vi "Home Screen.vi"() -> ()   [LabVIEW 2025]
doc: "Login"
uses:
  Host Globals/Global 1.vi
panel:
  out "Time":string
  out "User":string
  in  "Administration":bool
  in  "Audit Trail":bool
  in  "Exit":bool
  in  "HistoricalData":bool
  in  "ConfigurationMain":bool
  in  "Maintenance":bool
  in  "Test":bool
  # "Automated Testing of NVH Powertrain Lab"
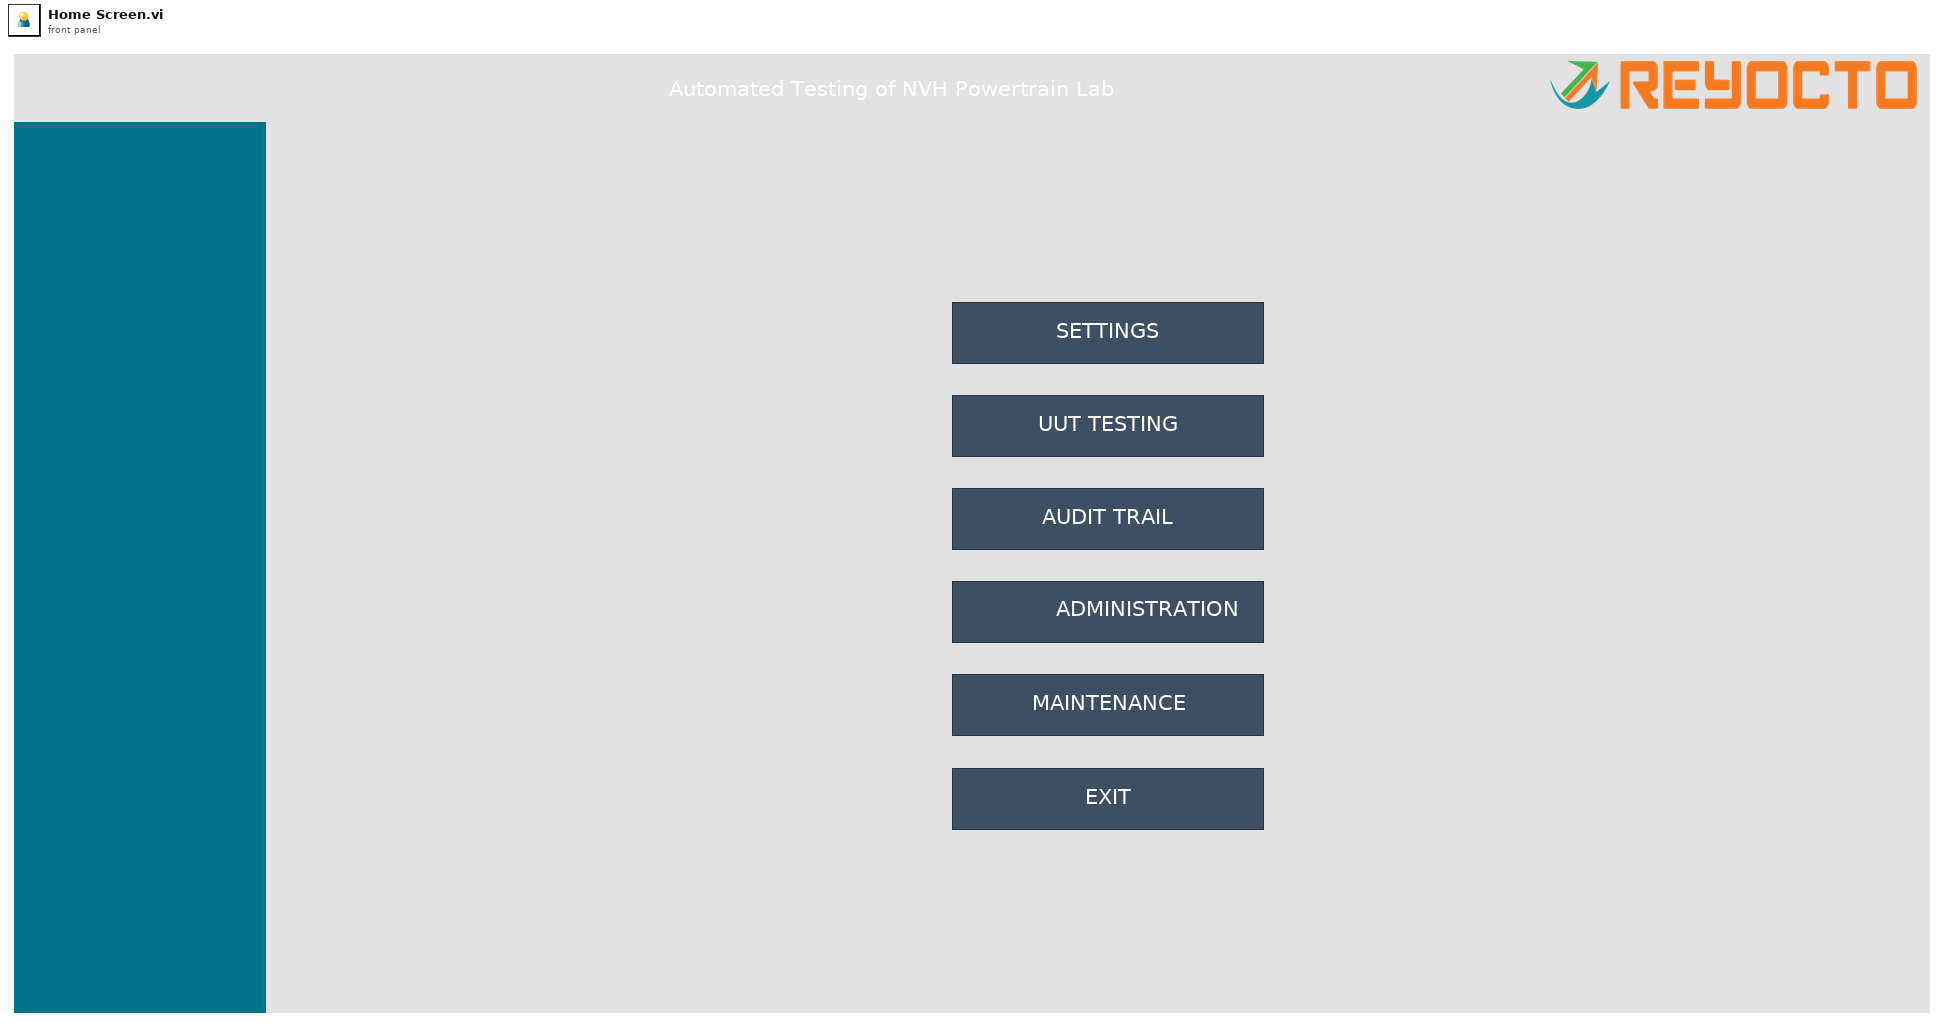
[diagram p1: front panel]
types:
  T1 = enum32{"Invalid", "Standard", "Closed", "Hidden", "Minimized", "Maximized"}
  T2 = enum32{"invalid app kind", "Development System", "Run Time System", "Student Edition", "Embedded LabVIEW", "Evaluation", "Custom"}
  T3 = cluster{"Core":cluster{"Current VI Reference":refnum<vi>, "Close Panel on Exit?":bool}, "VI Path":path, "Your string data":string}
  T4 = cluster{"Current VI Reference":refnum<vi>, "Close Panel on Exit?":bool}
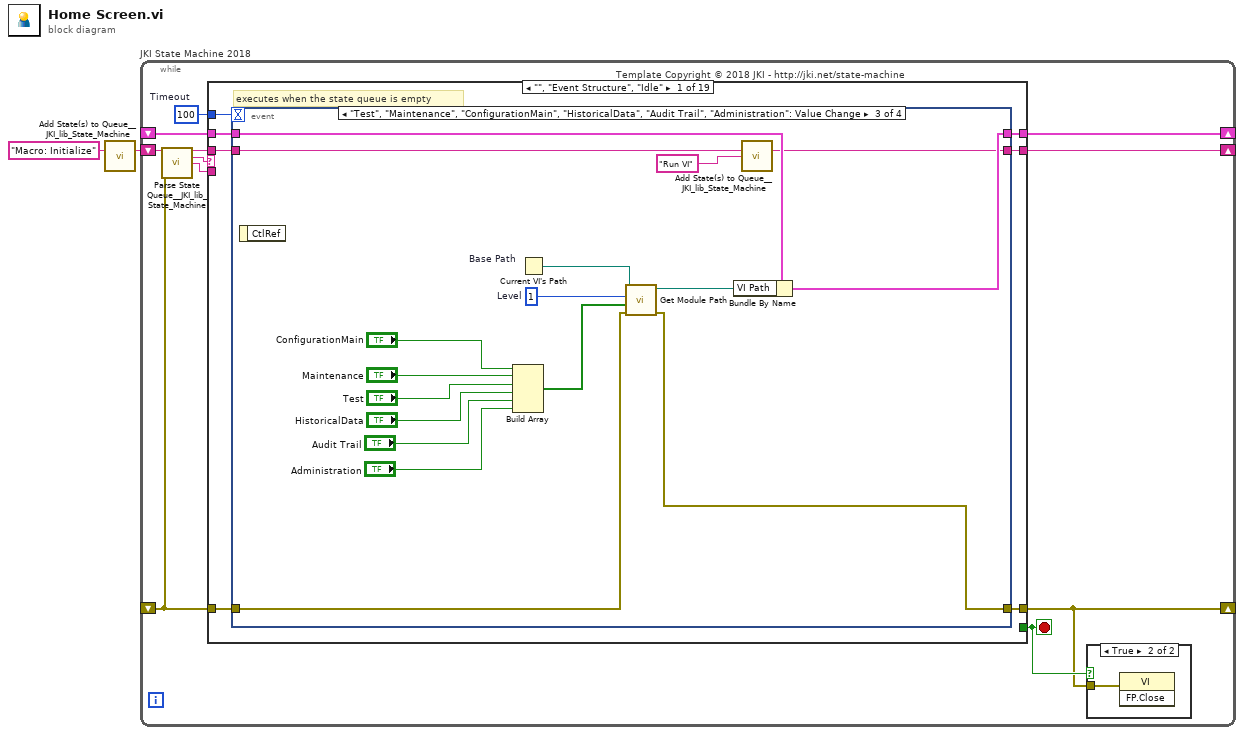
[diagram p0: block diagram]
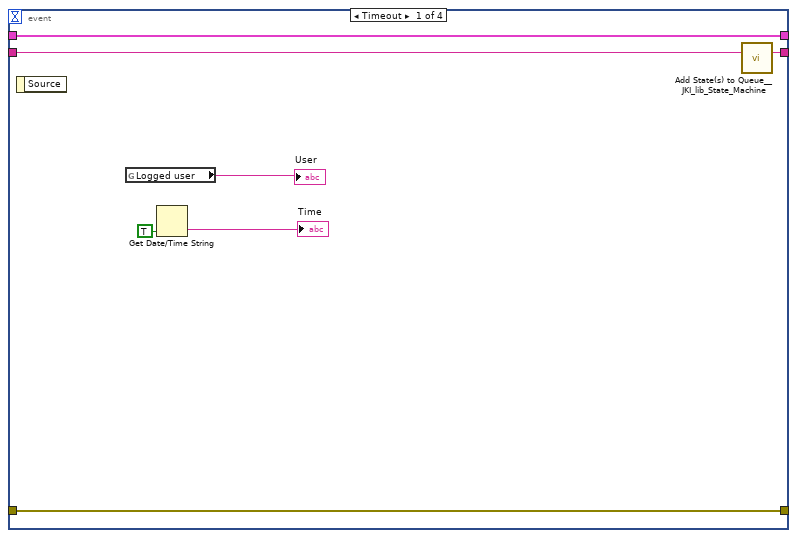
[diagram p3: hidden frame]
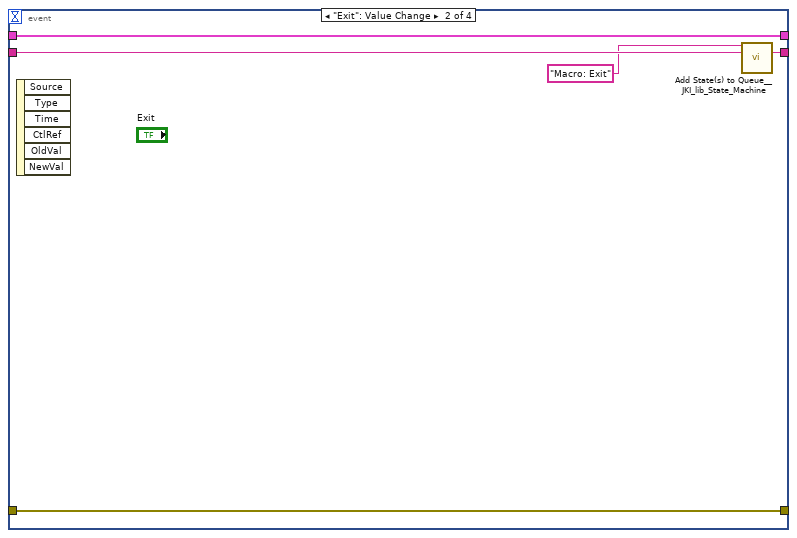
[diagram p4: hidden frame]
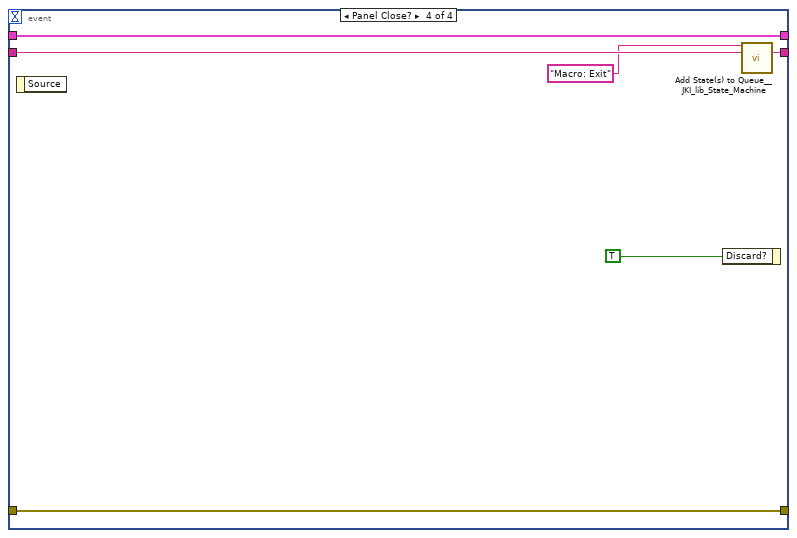
[diagram p5: hidden frame]
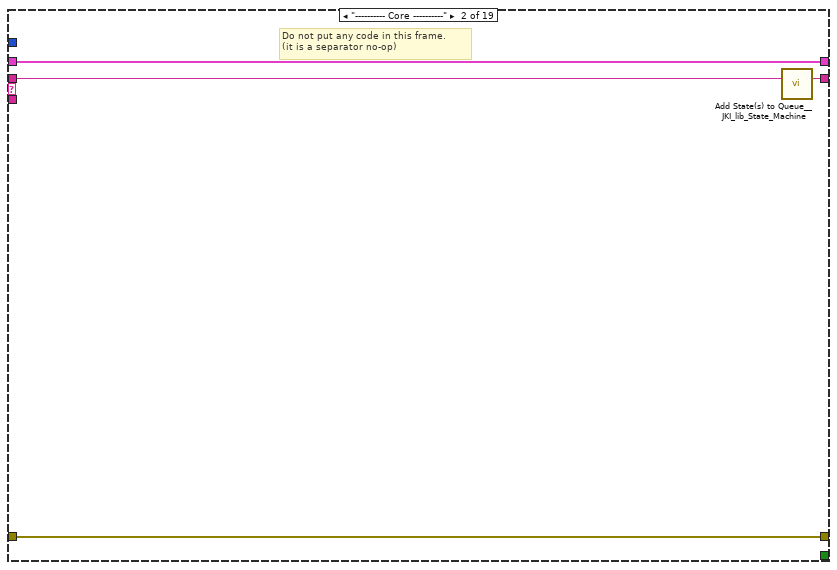
[diagram p6: hidden frame]
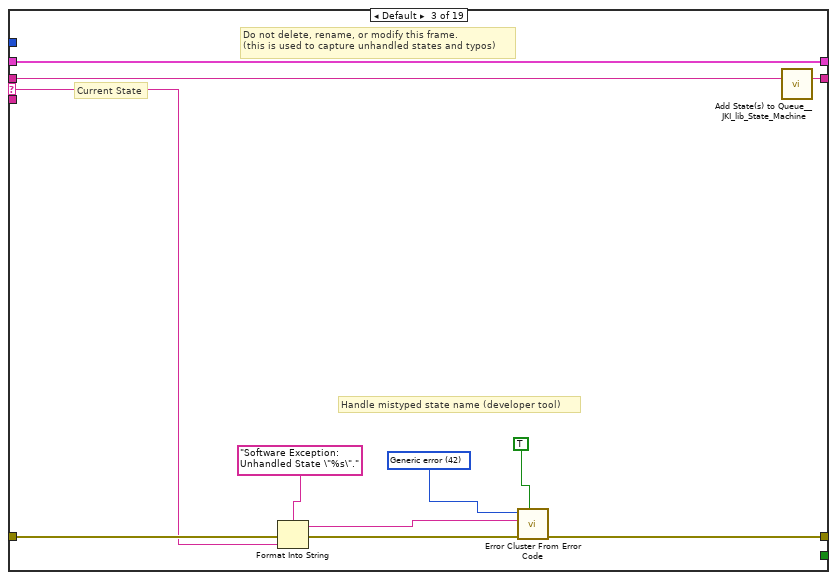
[diagram p7: hidden frame]
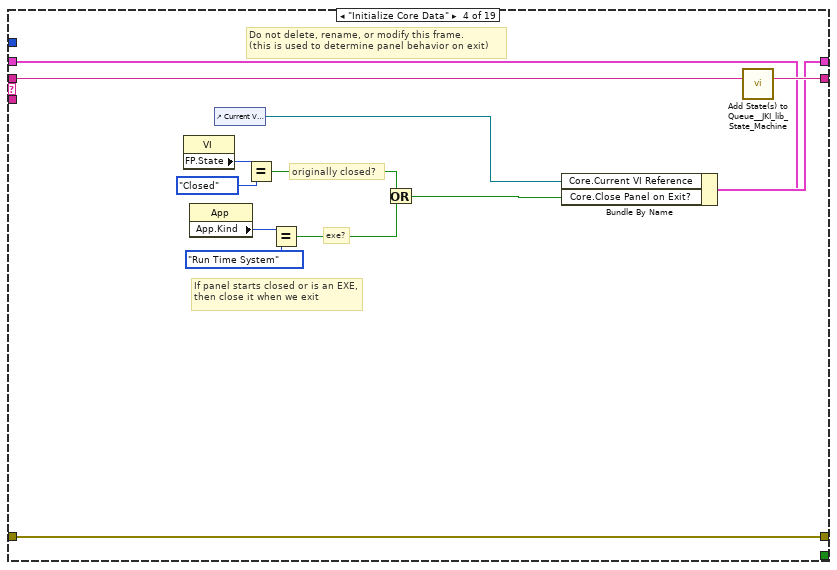
[diagram p8: hidden frame]
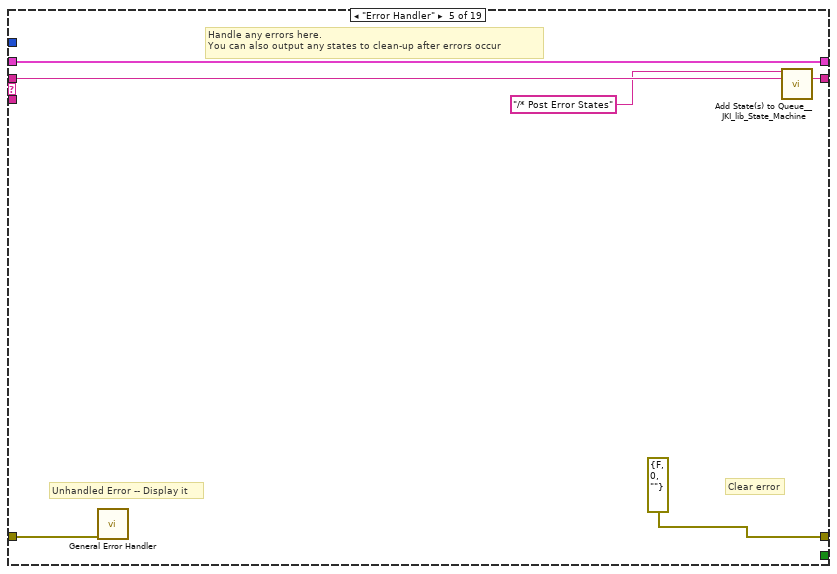
[diagram p9: hidden frame]
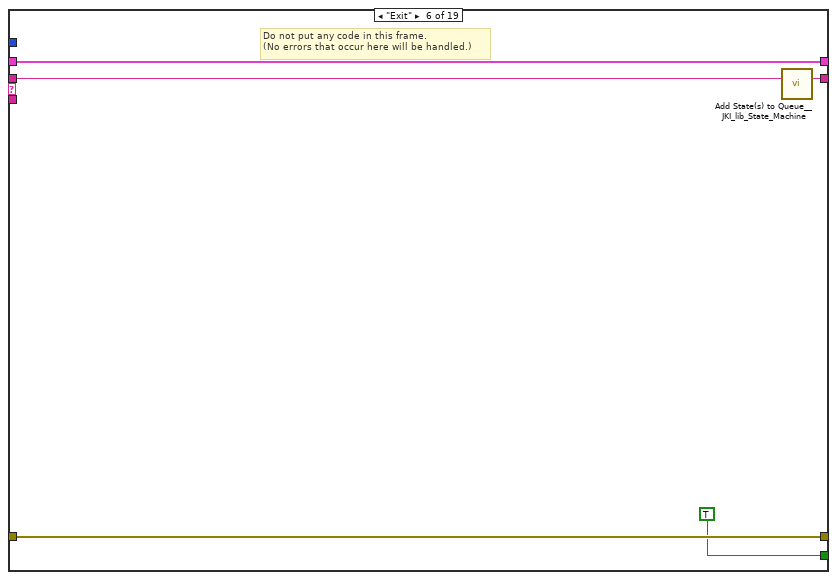
[diagram p10: hidden frame]
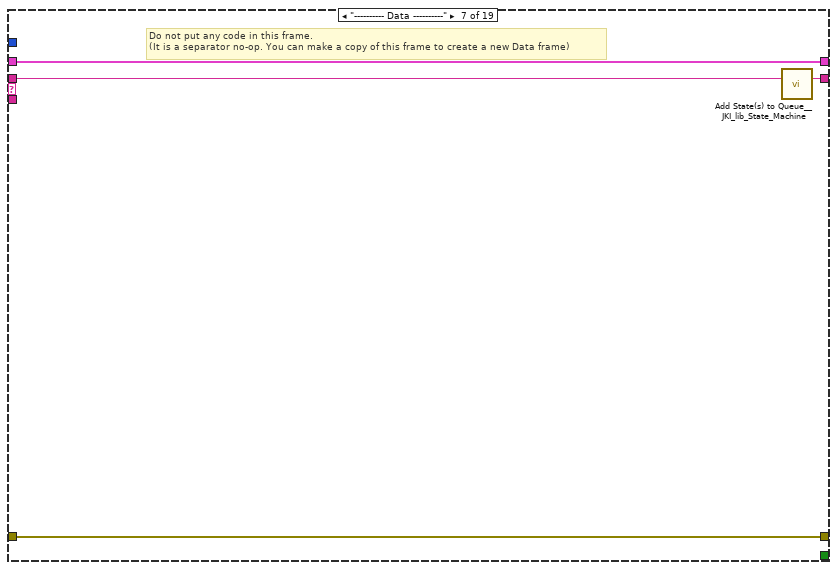
[diagram p11: hidden frame]
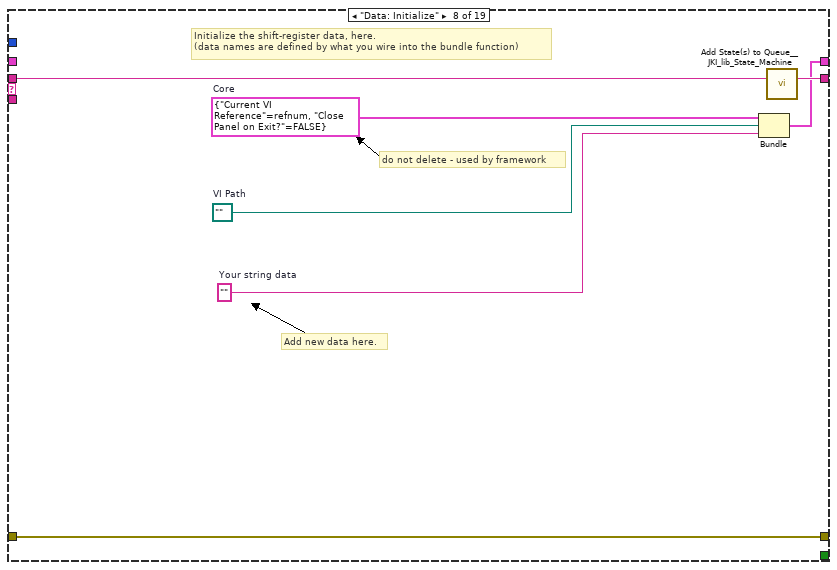
[diagram p12: hidden frame]
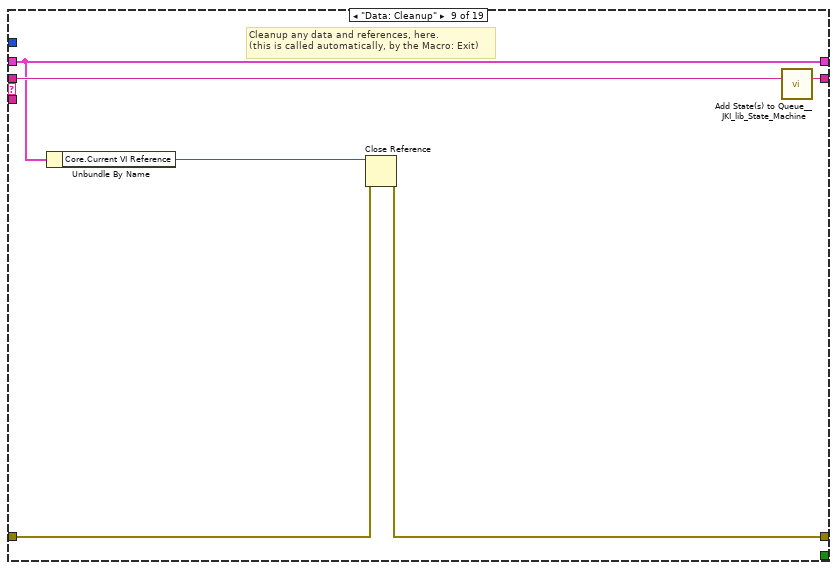
[diagram p13: hidden frame]
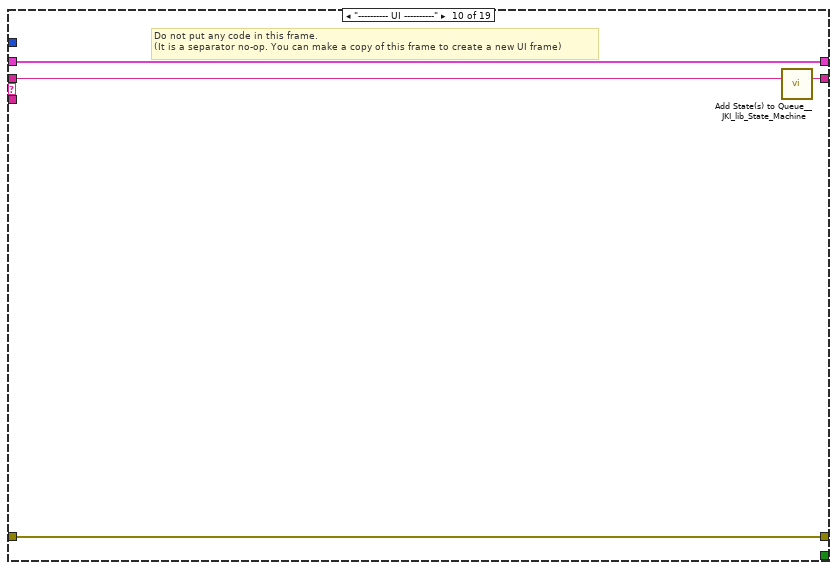
[diagram p14: hidden frame]
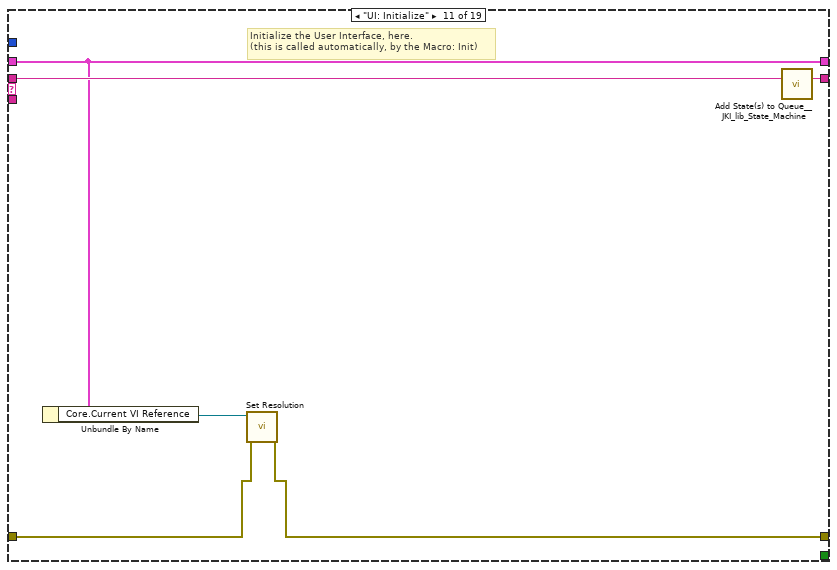
[diagram p15: hidden frame]
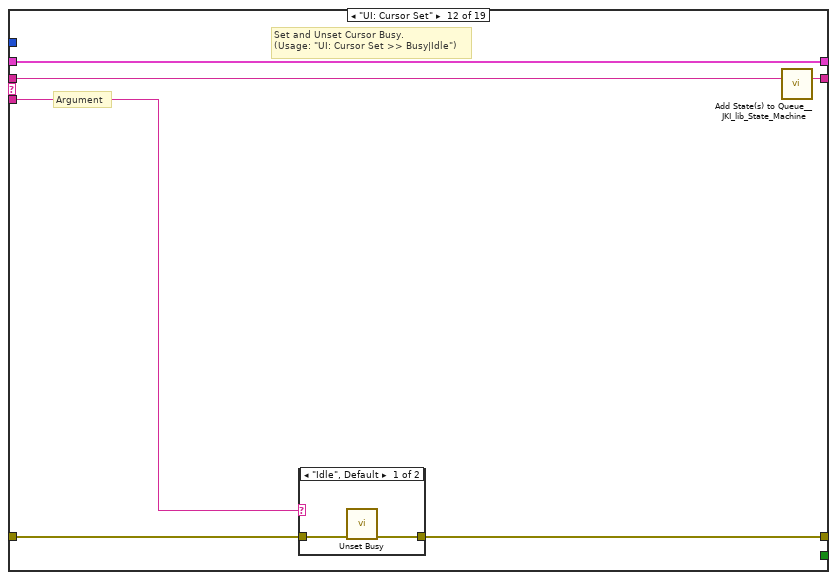
[diagram p16: hidden frame]
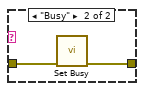
[diagram p17: hidden frame]
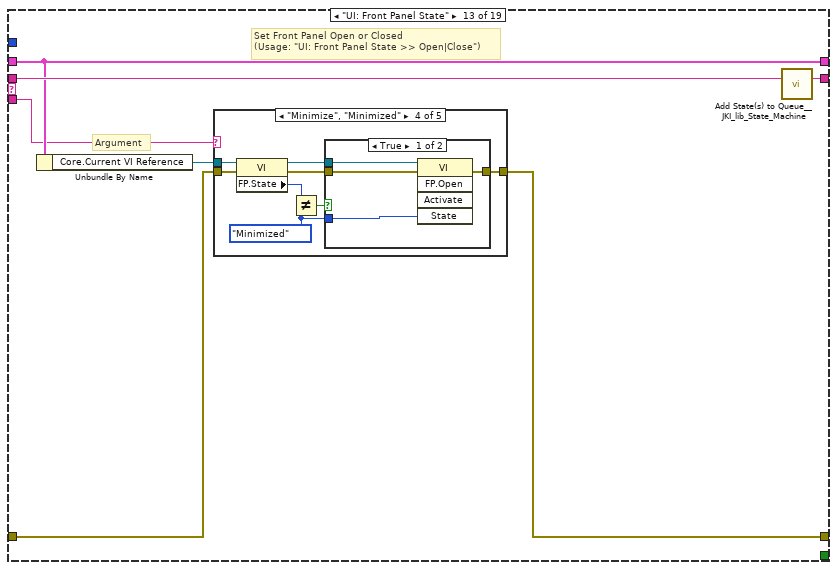
[diagram p18: hidden frame]
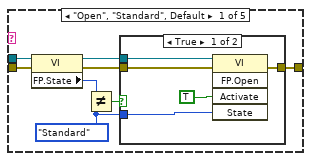
[diagram p19: hidden frame]
diagram:
  n1 = call <vilib>:"Add State(s) to Queue__JKI_lib_State_Machine.vi"("State(s) in (\"\")"="Macro: Initialize") -> ("States Out"=w2:string)  [unwired: 14 in]
  n2 = while "JKI State Machine 2018" {
    shift-right: [w8] -> _
    shift-left: _ -> [w7]
    shift-right: [w3] -> _
    shift-left: _ -> [w5]
    shift-right: [w9] -> _
    shift-left: w2 -> [w10]
    stop <- w4 stop-if-true
    w6 = 100  # Timeout
    # "Template Copyright © 2018 JKI - http://jki.net/state-machine"
    n3 = call <vilib>:"Parse State Queue__JKI_lib_State_Machine.vi"("State Queue"=w10, "Error In (no error)"=w5) -> ("Remaining States"=w12:string, "Current State"=w13:string, "Arguments"=w11:string)  [unwired: 11 in]
    n4 = case shown="\"\", \"Event Structure\", \"Idle\"" w13 {
      selector: w13 -> [_ _ w61 _ _ _ _ _ _ _ _ _ _ _ _ _ _ _ _]
      tunnel: w12 -> [w21 w60 w65 w84 w90 w95 w99 w106 w112 w116 w122 w128 w139 w208 w213 w223 w227 w240 w253]
      tunnel: w11 -> [_ _ _ _ _ _ _ _ _ _ _ w123 w133 _ _ _ _ _ _]
      tunnel: w7 -> [w19 w57 w63 w77 w87 w93 w96 _ w107 w113 w118 w126 w135 w205 w210 w220 w224 w237 w250]
      tunnel: [w18 w58 w67 w81 errorcluster {"status"=FALSE, "code"=0, "source"=""} ("error out") w92 w97 w103 w108 w114 w119 w124 w136 w206 w211 w221 w225 w229 w251] -> w3
      tunnel: w5 -> [w17 w58 w66 w81 w86 w92 w97 w103 w109 w114 w120 w125 w137 w206 w211 w221 w225 w238 w251]
      tunnel: [w20 w59 w64 w83 w89 w94 w98 w105 w111 w115 w121 w127 w138 w207 w212 w222 w226 w239 w252] -> w9
      tunnel: [_ _ _ _ _ TRUE _ _ _ _ _ _ _ _ _ _ _ w228 _] -> w4
      tunnel: [w16 w57 w63 w82 w87 w93 w96 w104 w107 w113 w118 w126 w135 w205 w210 w220 w224 w237 w250] -> w8
      tunnel: w6 -> [w15 _ _ _ _ _ _ _ _ _ _ _ _ _ _ _ _ _ _]
      frame "", "Event Structure", "Idle" {
        # "executes when the state queue is empty"
        n5 = event shown="[2] \"Test\", \"Maintenance\", \"ConfigurationMain\", \"HistoricalData\", \"Audit Trail\", \"Administration\": Value Change" {
          selector: _ -> [_ _ _ _]
          dyn-events: _ -> [_ _ _ _]
          timeout: w15 -> [_ _ _ _]
          tunnel: w21 -> [w28 w33 w39 w56]
          tunnel: [w27 w32 w40 w55] -> w20
          tunnel: w19 -> [w25 w30 w43 w53]
          tunnel: [w26 w31 w34 w54] -> w18
          tunnel: w17 -> [w26 w31 w45 w54]
          tunnel: [w25 w30 w42 w53] -> w16
          event Timeout {
            n6 = event-data() -> ()  [unwired: 1 in, 1 out]
            n7 = global read "Global 1.vi" "Logged user"() -> (→"User":string)
            n8 = Get Date/Time String(want seconds? (F)=TRUE) -> (time string=→"Time":string)  [unwired: 2 in, 1 out]
            n9 = call <vilib>:"Add State(s) to Queue__JKI_lib_State_Machine.vi"("State(s) in (\"\")"=w28) -> ("States Out"=w27:string)  [unwired: 14 in]
          }
          event "Exit": Value Change {
            n10 = event-data() -> ()  [unwired: 1 in, 6 out]
            n11 = call <vilib>:"Add State(s) to Queue__JKI_lib_State_Machine.vi"("State(s) in Front (\"\")"="Macro: Exit", "State(s) in (\"\")"=w33) -> ("States Out"=w32:string)  [unwired: 13 in]
          }
          event "Test", "Maintenance", "ConfigurationMain", "HistoricalData", "Audit Trail", "Administration": Value Change {
            w46 = 1  # Level
            n12 = event-data() -> ()  [unwired: 1 in, 1 out]
            n13 = Build Array("ConfigurationMain", "Maintenance", "Test", "HistoricalData", "Audit Trail", "Administration") -> (w44:bool[])
            n14 = Current VI's Path "Base Path"() -> (path=w47:path)
            n15 = call "Get Module Path.vi"("error in (no error)"=w45, "Array 2"=w44, "Level"=w46, "path"=w47) -> ("error out"=w34:errorcluster, "Selected Path"=w41:path)  [unwired: 5 in, 1 out]
            n16 = Bundle By Name(cluster=w43, "VI Path"=w41) -> (w42:T3)
            n17 = call <vilib>:"Add State(s) to Queue__JKI_lib_State_Machine.vi"("State(s) in (\"\")"=w39, "State(s) at Back (\"\")"="Run VI" ("State(s) at Back (\"\")")) -> ("States Out"=w40:string)  [unwired: 13 in]
          }
          event Panel Close? {
            n18 = event-data() -> ()  [unwired: 1 in, 1 out]
            n19 = event-data("Discard?"=TRUE) -> ()  [unwired: 1 in, 1 out]
            n20 = call <vilib>:"Add State(s) to Queue__JKI_lib_State_Machine.vi"("State(s) in Front (\"\")"="Macro: Exit", "State(s) in (\"\")"=w56) -> ("States Out"=w55:string)  [unwired: 13 in]
          }
        }
      }
      frame "---------- Core ----------" {
        # "Do not put any code in this frame.\n(it is a separator no-op)"
        n21 = call <vilib>:"Add State(s) to Queue__JKI_lib_State_Machine.vi"("State(s) in (\"\")"=w60) -> ("States Out"=w59:string)  [unwired: 14 in]
      }
      frame Default {
        w70 = 42 items=["No error", "Argument error", "Memory is full", "Out of zone", "End of file", "File already open", "Generic file I/O error", "File not found", "File permission error", "Disk is full", "Duplicate path", "Too many files open", "System feature not enabled", "Resource file not found", "Cannot add resource", "Resource not found", "Image not found", "Image memory error", "Pen does not exist", "Config type invalid", "Config token not found", "Config parse error", "Config memory error", "Bad external code format", "Bad external code offset", "External code not present", "Null window", "Destroy window error", "Null menu", "Print aborted", "Bad print record", "Print driver error", "Windows error during printing", "Memory error during printing", "Print dialog error", "Generic print error", "Invalid device refnum", "Device not found", "Device parameter error", "Device unit error", "Cannot open device", "Device call aborted", "Generic error", "Cancelled by user", "Object ID too low", "Object ID too high", "Object not in heap", "Unknown heap", "Unknown object (invalid DefProc)", "Unknown object (DefProc not in table)", "Message out of range", "Invalid (null) method", "Unknown message", "Manager call not supported", "Bad address", "Network operation in progress", "Network operation timed out", "Connection is busy", "Network attribute not supported", "Network error", "Address in use", "System out of memory", "Connection aborted", "Connection refused", "Not connected", "Already connected", "Connection closed", "Initialization error (interapplication manager)", "Bad occurrence", "Wait on unbound occurrence handler", "Occurrence queue overflow", "Datalog type conflict", "Unused", "Unrecognized type (interapplication manager)", "Memory corrupt", "Failed to make temporary DLL", "Old CIN version", "Drag socket not found", "Failed to load drop-object", "Failed to register OLE object", "Failed to release OLE object", "Format specifier type mismatch", "Unknown format specifier", "Too few format specifiers", "Too many format specifiers", "Scan failed", "Newer CIN version", "Error converting to variant", "Runtime menu error", "Password tampered", "Variant attribute not found", "Incompatible variant data type", "Event data is not available", "Event Store is not present", "Occurrence is not found", "Event Queue is not created", "Event info is not available", "Refnum passed is NULL", "Error retrieving Class GUID", "Error retrieving CoClass GUID", "Error retrieving TypeLib GUID.", "Bad built application magic bytes.", "Specific driver is different from the specific driver associated with the Logical Name.", "There is no session opened to the class driver.", "Max Error", "MAX - Error with config objects", "MAX - Error loading configuration", "MAX - Group not supported"]
        # "Current State"
        # "Do not delete, rename, or modify this frame.\n(this is used to capture unhandled states and typos)"
        # "Handle mistyped state name (developer tool)"
        n22 = Format Into String(format string="Software Exception: Unhandled State \"%s\"." ("message"), error in=w66, w61) -> (resulting string=w69:string, error out=w68:errorcluster)  [unwired: 1 in]
        n23 = call <vilib>:"Error Cluster From Error Code.vi"("show call chain? (False)"=TRUE, "error in (no error)"=w68, "error message (\"\")"=w69, "error code (0)"=w70) -> ("error out"=w67:errorcluster)  [unwired: 5 in]
        n24 = call <vilib>:"Add State(s) to Queue__JKI_lib_State_Machine.vi"("State(s) in (\"\")"=w65) -> ("States Out"=w64:string)  [unwired: 14 in]
      }
      frame "Initialize Core Data" {
        # "Do not delete, rename, or modify this frame.\n(this is used to determine panel behavior on exit)"
        # "originally closed?"
        # "exe?"
        # "If panel starts closed or is an EXE, then close it when we exit"
        n25 = property class="VI"() -> ("FP.State"=w74:T1)  [unwired: 2 in, 2 out]
        n26 = property class="App"() -> ("App.Kind"=w80:T2)  [unwired: 2 in, 2 out]
        n27 = control-ref of="Current VI Reference"() -> (w75:refnum<vi>)
        n28 = Equal?(x=w74, y=T1."Closed" ("Front Panel Window:State")) -> (x = y?=w72:bool)
        n29 = Equal?(x=w80, y=T2."Run Time System" ("Application:Kind")) -> (x = y?=w78:bool)
        n30 = Or(x=w72, y=w78) -> (x .or. y?=w76:bool)
        n31 = Bundle By Name(cluster=w77, "Core.Current VI Reference"=w75, "Core.Close Panel on Exit?"=w76) -> (w82:T3)
        n32 = call <vilib>:"Add State(s) to Queue__JKI_lib_State_Machine.vi"("State(s) in (\"\")"=w84) -> ("States Out"=w83:string)  [unwired: 14 in]
      }
      frame "Error Handler" {
        # "Unhandled Error -- Display it"
        # "Handle any errors here.\nYou can also output any states to clean-up after errors occur"
        # "Clear error"
        n33 = call <vilib>:"General Error Handler.vi"("error in (no error)"=w86) -> ()  [unwired: 10 in, 5 out]
        n34 = call <vilib>:"Add State(s) to Queue__JKI_lib_State_Machine.vi"("State(s) in Front (\"\")"="/* Post Error States", "State(s) in (\"\")"=w90) -> ("States Out"=w89:string)  [unwired: 13 in]
      }
      frame "Exit" {
        # "Do not put any code in this frame.\n(No errors that occur here will be handled.)"
        n35 = call <vilib>:"Add State(s) to Queue__JKI_lib_State_Machine.vi"("State(s) in (\"\")"=w95) -> ("States Out"=w94:string)  [unwired: 14 in]
      }
      frame "---------- Data ----------" {
        # "Do not put any code in this frame.\n(It is a separator no-op. You can make a copy of this frame to create a new Data frame)"
        n36 = call <vilib>:"Add State(s) to Queue__JKI_lib_State_Machine.vi"("State(s) in (\"\")"=w99) -> ("States Out"=w98:string)  [unwired: 14 in]
      }
      frame "Data: Initialize" {
        w100 = path ""  # VI Path
        w101 = T4 {"Current VI Reference"=refnum, "Close Panel on Exit?"=FALSE}  # Core
        w102 = ""  # Your string data
        # "do not delete - used by framework"
        # "Add new data here."
        # "Initialize the shift-register data, here.\n(data names are defined by what you wire into the bundle function)"
        n37 = Bundle("Core"=w101, "VI Path"=w100, "Your string data"=w102) -> (w104:T3)  [unwired: 1 in]
        n38 = call <vilib>:"Add State(s) to Queue__JKI_lib_State_Machine.vi"("State(s) in (\"\")"=w106) -> ("States Out"=w105:string)  [unwired: 14 in]
      }
      frame "Data: Cleanup" {
        # "Cleanup any data and references, here.\n(this is called automatically, by the Macro: Exit)"
        n39 = Unbundle By Name(w107) -> ("Core.Current VI Reference"=w110:refnum<vi>)
        n40 = Close Reference(reference=w110, error in (no error)=w109) -> (error out=w108:errorcluster)
        n41 = call <vilib>:"Add State(s) to Queue__JKI_lib_State_Machine.vi"("State(s) in (\"\")"=w112) -> ("States Out"=w111:string)  [unwired: 14 in]
      }
      frame "---------- UI ----------" {
        # "Do not put any code in this frame.\n(It is a separator no-op. You can make a copy of this frame to create a new UI frame)"
        n42 = call <vilib>:"Add State(s) to Queue__JKI_lib_State_Machine.vi"("State(s) in (\"\")"=w116) -> ("States Out"=w115:string)  [unwired: 14 in]
      }
      frame "UI: Initialize" {
        # "Initialize the User Interface, here.\n(this is called automatically, by the Macro: Init)"
        n43 = Unbundle By Name(w118) -> ("Core.Current VI Reference"=w117:refnum<vi>)
        n44 = call "Set Resolution.vi"("error in (no error)"=w120, "VI in"=w117) -> ("error out"=w119:errorcluster)  [unwired: 8 in, 1 out]
        n45 = call <vilib>:"Add State(s) to Queue__JKI_lib_State_Machine.vi"("State(s) in (\"\")"=w122) -> ("States Out"=w121:string)  [unwired: 14 in]
      }
      frame "UI: Cursor Set" {
        # "Argument"
        # "Set and Unset Cursor Busy.\n(Usage: \"UI: Cursor Set >> Busy|Idle\")"
        n46 = case shown="\"Idle\", Default" w123 {
          tunnel: w125 -> [w130 w132]
          tunnel: [w129 w131] -> w124
          frame "Idle", Default {
            n47 = call <vilib>:"Unset Busy.vi"("error in (no error)"=w130) -> ("error out"=w129:errorcluster)  [unwired: 10 in]
          }
          frame "Busy" {
            n48 = call <vilib>:"Set Busy.vi"("error in (no error)"=w132) -> ("error out"=w131:errorcluster)  [unwired: 9 in, 1 out]
          }
        }
        n49 = call <vilib>:"Add State(s) to Queue__JKI_lib_State_Machine.vi"("State(s) in (\"\")"=w128) -> ("States Out"=w127:string)  [unwired: 14 in]
      }
      frame "UI: Front Panel State" {
        # "Argument"
        # "Set Front Panel Open or Closed\n(Usage: \"UI: Front Panel State >> Open|Close\")"
        n50 = Unbundle By Name(w135) -> ("Core.Current VI Reference"=w134:refnum<vi>)
        n51 = case shown="\"Minimize\", \"Minimized\"" w133 {
          tunnel: w137 -> [w145 w160 w171 w184 w197]
          tunnel: [w147 w161 w173 w186 w199] -> w136
          tunnel: w134 -> [w146 w158 w172 w185 w198]
          frame "Open", "Standard", Default {
            w140 = T1."Standard" ("State")
            n52 = property class="VI"(reference=w146, error in=w145) -> (reference out=w143:refnum<vi>, error out=w144:errorcluster, "FP.State"=w142:T1)
            n53 = Not Equal?(x=w142, y=w140) -> (x != y?=w141:bool)
            n54 = case shown="True" w141 {
              tunnel: [w151 w153] -> w147
              tunnel: w144 -> [w150 w153]
              tunnel: w143 -> [w149 _]
              tunnel: w140 -> [w148 _]
              frame True {
                n55 = invoke class="VI" method="FP.Open"(reference=w149, error in=w150, "Activate"=TRUE, "State"=w148) -> (error out=w151:errorcluster)  [unwired: 1 in, 4 out]
              }
              frame False {
              }
            }
          }
          frame "Close", "Closed" {
            n56 = property class="VI"(reference=w158, error in=w160) -> (reference out=w157:refnum<vi>, error out=w159:errorcluster, "FP.State"=w155:T1)
            n57 = Not Equal?(x=w155, y=T1."Closed" ("Front Panel Window:State")) -> (x != y?=w154:bool)
            n58 = case shown="True" w154 {
              tunnel: [w162 w165] -> w161
              tunnel: w159 -> [w162 w164]
              tunnel: w157 -> [_ w163]
              frame False {
              }
              frame True {
                n59 = invoke class="VI" method="FP.Close"(reference=w163, error in=w164) -> (error out=w165:errorcluster)  [unwired: 1 in, 2 out]
              }
            }
          }
          frame "Hidden", "Hide" {
            w166 = T1."Hidden" ("State")
            n60 = property class="VI"(reference=w172, error in=w171) -> (reference out=w169:refnum<vi>, error out=w170:errorcluster, "FP.State"=w168:T1)
            n61 = Not Equal?(x=w168, y=w166) -> (x != y?=w167:bool)
            n62 = case shown="True" w167 {
              tunnel: [w177 w178] -> w173
              tunnel: w170 -> [w176 w178]
              tunnel: w169 -> [w175 _]
              tunnel: w166 -> [w174 _]
              frame True {
                n63 = invoke class="VI" method="FP.Open"(reference=w175, error in=w176, "State"=w174) -> (error out=w177:errorcluster)  [unwired: 2 in, 4 out]
              }
              frame False {
              }
            }
          }
          frame "Minimize", "Minimized" {
            w179 = T1."Minimized" ("State")
            n64 = property class="VI"(reference=w185, error in=w184) -> (reference out=w182:refnum<vi>, error out=w183:errorcluster, "FP.State"=w181:T1)
            n65 = Not Equal?(x=w181, y=w179) -> (x != y?=w180:bool)
            n66 = case shown="True" w180 {
              tunnel: [w190 w191] -> w186
              tunnel: w183 -> [w189 w191]
              tunnel: w182 -> [w188 _]
              tunnel: w179 -> [w187 _]
              frame True {
                n67 = invoke class="VI" method="FP.Open"(reference=w188, error in=w189, "State"=w187) -> (error out=w190:errorcluster)  [unwired: 2 in, 4 out]
              }
              frame False {
              }
            }
          }
          frame "Maximize", "Maximized" {
            w192 = T1."Maximized" ("State")
            n68 = property class="VI"(reference=w198, error in=w197) -> (reference out=w195:refnum<vi>, error out=w196:errorcluster, "FP.State"=w194:T1)
            n69 = Not Equal?(x=w194, y=w192) -> (x != y?=w193:bool)
            n70 = case shown="True" w193 {
              tunnel: [w203 w204] -> w199
              tunnel: w196 -> [w202 w204]
              tunnel: w195 -> [w201 _]
              tunnel: w192 -> [w200 _]
              frame True {
                n71 = invoke class="VI" method="FP.Open"(reference=w201, error in=w202, "State"=w200) -> (error out=w203:errorcluster)  [unwired: 2 in, 4 out]
              }
              frame False {
              }
            }
          }
        }
        n72 = call <vilib>:"Add State(s) to Queue__JKI_lib_State_Machine.vi"("State(s) in (\"\")"=w139) -> ("States Out"=w138:string)  [unwired: 14 in]
      }
      frame "---------- Macro ----------" {
        # "Do not put any code in this frame.\n(It is a separator no-op. You can make a copy of this frame to create a new Macro frame)"
        n73 = call <vilib>:"Add State(s) to Queue__JKI_lib_State_Machine.vi"("State(s) in (\"\")"=w208) -> ("States Out"=w207:string)  [unwired: 14 in]
      }
      frame "Macro: Initialize" {
        w209 = "Data: Initialize\nInitialize Core Data\nUI: Initialize\nUI: Front Panel State >> Open"  # Data: Initialize Initialize Core Data UI: Initialize UI: Front Panel State >> Open
        # "Initialization Macro\n(This is called once, when the VI starts)"
        n74 = call <vilib>:"Add State(s) to Queue__JKI_lib_State_Machine.vi"("State(s) in Front (\"\")"=w209, "State(s) in (\"\")"=w213) -> ("States Out"=w212:string)  [unwired: 13 in]
      }
      frame "Macro: Exit" {
        # "Exit Macro\n(This is called once, when the VI exits)"
        n75 = Unbundle By Name(w220) -> ("Core.Close Panel on Exit?"=w219:bool)
        n76 = Select(t="UI: Front Panel State >> Close", s=w219, f="") -> (s? t:f=w216:string)
        n77 = call <vilib>:"Add State(s) to Queue__JKI_lib_State_Machine.vi"("State(s) in (\"\")"=w216, "State(s) at Back (\"\")"="Data: Cleanup\nExit") -> ("States Out"=w214:string)  [unwired: 13 in]
        n78 = call <vilib>:"Add State(s) to Queue__JKI_lib_State_Machine.vi"("State(s) in Front (\"\")"=w214, "State(s) in (\"\")"=w223) -> ("States Out"=w222:string)  [unwired: 13 in]
      }
      frame "---------- New Category ----------" {
        # "Template Separator\n(You can make a copy of, or modify, this frame)"
        n79 = call <vilib>:"Add State(s) to Queue__JKI_lib_State_Machine.vi"("State(s) in (\"\")"=w227) -> ("States Out"=w226:string)  [unwired: 14 in]
      }
      frame "Run VI" {
        n80 = Unbundle By Name(w237) -> ("VI Path"=w234:path)
        n81 = call "Run VI Dynamically2.vi"("error in (no error)"=w238, "Show FP?"=TRUE, "Vi Path"=w234) -> ("error out"=w235:errorcluster)  [unwired: 7 in, 1 out]
        n82 = Strip Path(path=w234) -> (stripped path=w230:path, name=w232:string)
        n83 = Equal?(x=w232, y="Main_CS_Auto.vi" ("name or relative path")) -> (x = y?=w231:bool)
        n84 = case shown="True" w231 {
          tunnel: w235 -> [w242 w246]
          tunnel: [w242 w245] -> w229
          tunnel: w230 -> [_ w244]
          tunnel: [FALSE ("Show FP?") TRUE ("Show FP?")] -> w228
          frame False {
          }
          frame True {
            n85 = Build Path(base path=w244, name or relative path="Data Monitor_Auto.vi") -> (appended path=w247:path)
            n86 = call "Run VI Dynamically2.vi"("error in (no error)"=w246, "Show FP?"=TRUE, "Vi Path"=w247) -> ("error out"=w245:errorcluster)  [unwired: 7 in, 1 out]
          }
        }
        n87 = call <vilib>:"Add State(s) to Queue__JKI_lib_State_Machine.vi"("State(s) in (\"\")"=w240) -> ("States Out"=w239:string)  [unwired: 14 in]
      }
      frame "New Category: 2" {
        # "Your code here.\n(You can make a copy of, or modify, this frame)"
        n88 = call <vilib>:"Add State(s) to Queue__JKI_lib_State_Machine.vi"("State(s) in (\"\")"=w253) -> ("States Out"=w252:string)  [unwired: 14 in]
      }
    }
    n89 = case shown="True" w4 {
      tunnel: w3 -> [_ w14]
      frame False {
      }
      frame True {
        n90 = invoke class="VI" method="FP.Close"(error in=w14) -> ()  [unwired: 2 in, 3 out]
      }
    }
  }
